vi "Read Rules Parser Parameters.vi"(11 "CDependencyInspection in":refnum<class "CDependencyInspection.lvclass">) -> (1 "Parameters":string, 3 "CDependencyInspection out":refnum<class "CDependencyInspection.lvclass">)   [LabVIEW 2020, in "DependencyInspection.lvlib" / "CDependencyInspection.lvclass"]
uses:
  CDependencyInspection.lvclass
  CDependencyInspection.lvclass/CDependencyInspection.ctl
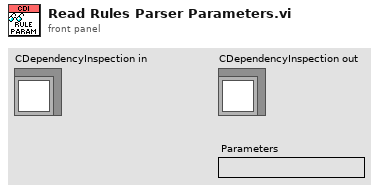
[diagram p1: front panel]
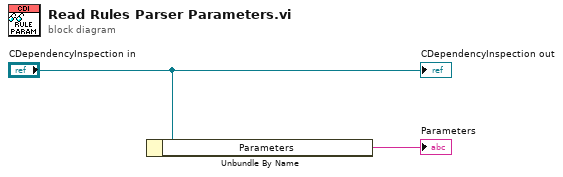
[diagram p0: block diagram]
diagram:
  n1 = Unbundle By Name("CDependencyInspection in") -> ("Parameters"=→"Parameters":string)
  "CDependencyInspection out" <- "CDependencyInspection in"
